vi "Calling.vi"(7 "Actor in":refnum<class "Actor.lvclass">, 10 "Msg Attributes":T1 {"Teller"."Absolute Time" format="%<%x %.3X>T"}) -> (0 "Error out":errorcluster, 5 "Actor out":refnum<class "Actor.lvclass">)   [LabVIEW 2020, in "jettl.lvlib"]
uses:
  jettl.lvlib
  Msg/Msg.lvclass
  Msg Input/Msg Input.lvclass
  Msg Output/Msg Output.lvclass
  Actor/Actor.lvclass
  Relation.ctl
  Teller.ctl
  Msg Attributes.ctl
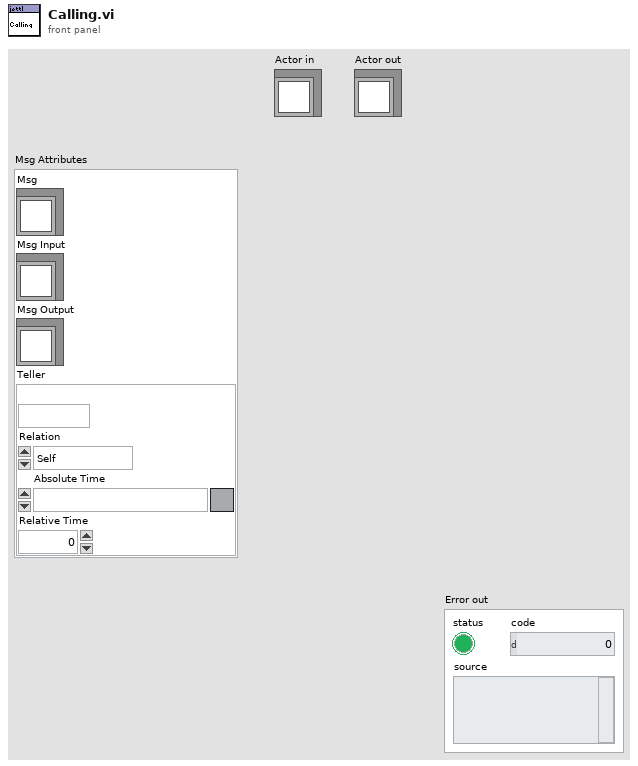
[diagram p1: front panel]
types:
  T1 = typedef "jettl.lvlib/Msg Attributes.ctl" = cluster{"Msg":refnum<class "Msg.lvclass">, "Msg Input":refnum<class "Msg Input.lvclass">, "Msg Output":refnum<class "Msg Output.lvclass">, "Teller":T2}
  T2 = typedef "jettl.lvlib/Teller.ctl" = cluster{"Alias":string, "Relation":T3, "Absolute Time":timestamp, "Relative Time":dbl}
  T3 = typedef "jettl.lvlib/Relation.ctl" = enum16{"Self", "Parent", "Child"}
  T4 = typedef "jettl.lvlib/Actor Attributes.ctl" = cluster{"Unified Layer":T5, "Root":bool, "Alias":string, "UID":i32, "Transport":refnum<user-event>, "Address":refnum<event-registration>, "This VI":refnum<vi>}
  T5 = typedef "jettl.lvlib/Unified Layer.ctl" = cluster{"Msgs":T6, "Leaf":bool}
  T6 = typedef "jettl.lvlib/Msgs.ctl" = set{refnum<class "Msg.lvclass">}
  T7 = typedef "jettl.lvlib/Msg Attributes.ctl" = cluster{"Msg":refnum<class "Msg.lvclass">, "Msg Input":refnum<class "Msg Input.lvclass">, "Msg Output":refnum<class "Msg Output.lvclass">, "Teller":T8}
  T8 = typedef "jettl.lvlib/Teller.ctl" = cluster{"Relation":T3, "Absolute Time":timestamp, "Relative Time":dbl, "Alias":string}
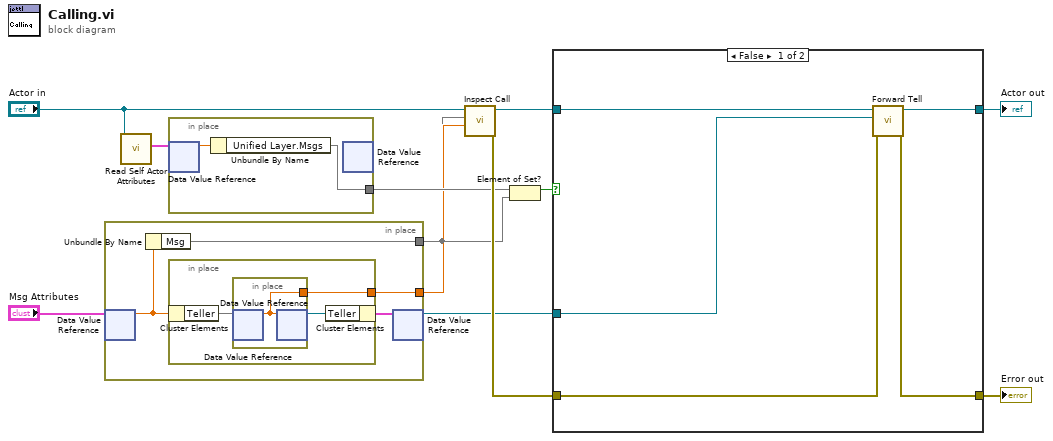
[diagram p0: block diagram]
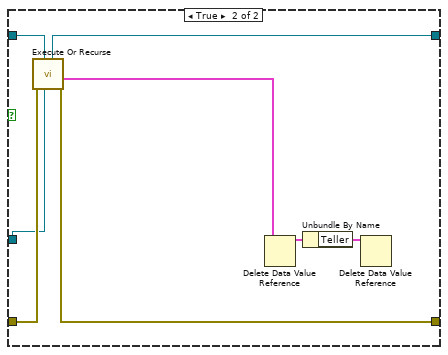
[diagram p2: hidden frame]
diagram:
  n1 = in-place {
    in-place-border: [w15] -> w3
    in-place-border: [w13] -> w2
    n2 = in-place-dvr #1("Msg Attributes") -> (w14:dbl)  [unwired: 1 out]
    n3 = Unbundle By Name(w14) -> ("Msg"=w13)
    n4 = in-place {
      in-place-border: [w17] -> w15
      n5 = in-place-cluster #2(w14) -> ("Teller"=w19)
      n6 = in-place {
        in-place-border: [w20] -> w17
        n7 = in-place-dvr #3(w19) -> (w20:dbl)  [unwired: 1 out]
        n8 = in-place-dvr #3(w20) -> (w18:refnum<data-value>)  [unwired: 1 out]
      }
      n9 = in-place-cluster #2("Teller"=w18) -> (w16:cluster{})
    }
    n10 = in-place-dvr #1(w16) -> (w4:refnum<data-value>)  [unwired: 1 out]
  }
  n11 = call-dynamic "Read Self Actor Attributes.vi"("Actor in"="Actor in") -> ("Self Actor Attributes"=w9:T4)  [unwired: 10 in]
  n12 = in-place {
    in-place-border: [w21] -> w8
    n13 = in-place-dvr #4(w9) -> (w22:dbl)  [unwired: 1 out]
    n14 = Unbundle By Name(w22) -> ("Unified Layer.Msgs"=w21)
    n15 = in-place-dvr #4() -> ()  [unwired: 1 in, 2 out]
  }
  n16 = call-dynamic "Inspect Call.vi"("Teller"=w3, "Msg"=w2, "Actor in"="Actor in") -> ("Error out"=w10:errorcluster, "Actor out"=w7:refnum<class "Actor.lvclass">)  [unwired: 7 in]
  n17 = Element of Set?(10:w2, 11:w8) -> (3:w6:bool)
  n18 = case shown="False" w6 {
    tunnel: [w26 w35] -> w12
    tunnel: [w24 w34] -> w11
    tunnel: w7 -> [w27 w33]
    tunnel: w10 -> [w25 w32]
    tunnel: w4 -> [w23 w31]
    frame False {
      n19 = call-dynamic "Forward Tell.vi"("Error in"=w25, "Msg Attributes"=w23, "Actor in"=w27) -> ("Error out"=w24:errorcluster, "Actor out"=w26:refnum<class "Actor.lvclass">)  [unwired: 7 in]
    }
    frame True {
      n20 = call "Execute Or Recurse.vi"("Msg Attributes in"=w31, "Actor in"=w33, "Error in"=w32) -> ("Error out"=w34:errorcluster, "Msg Attributes out"=w28:T1, "Actor out"=w35:refnum<class "Actor.lvclass">)  [unwired: 6 in]
      n21 = Delete Data Value Reference(data value reference=w28) -> (data value=w30:T7)  [unwired: 1 in, 1 out]
      n22 = Unbundle By Name(w30) -> ("Teller"=w29:T8)
      n23 = Delete Data Value Reference(data value reference=w29) -> ()  [unwired: 1 in, 2 out]
    }
  }
  "Actor out" <- w12
  "Error out" <- w11
